vi "getVariableStatus.vi"(0 "Controller in":refnum<class "_Controller.lvclass">, 2 "var_number":u16, 5 "error in (no error)":errorcluster) -> (14 "Controller out":refnum<class "_Controller.lvclass">, 16 "var_value":string, 19 "error out":errorcluster)   [LabVIEW 2020, in "classes.lvlib" / "_Controller.lvclass"]
doc: "Retrieves the Variable Value (output) at the given Variable Number (input)\n\nProduced By:\n\n<B>Kod Integrations, LLC</B>\n4835 Marianne Drive\nMount Airy, MD 21771\nhttp://www.kodintegrations.com\nemail: info@kodintegrations.com\nphone: (240) 687-1288"
uses:
  _Controller.lvclass
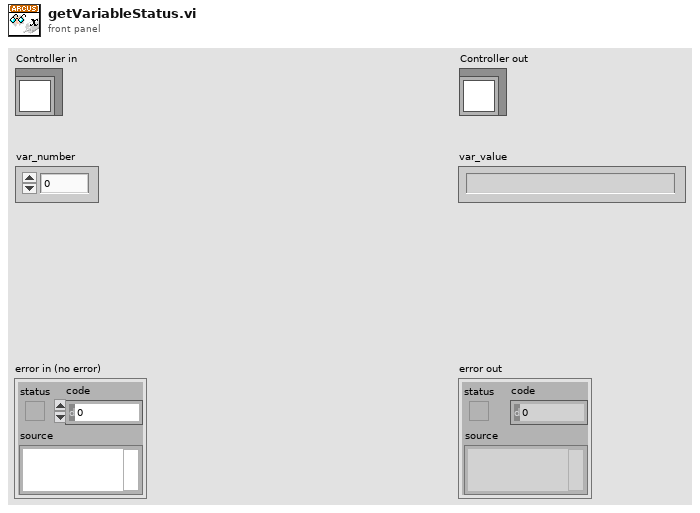
[diagram p1: front panel]
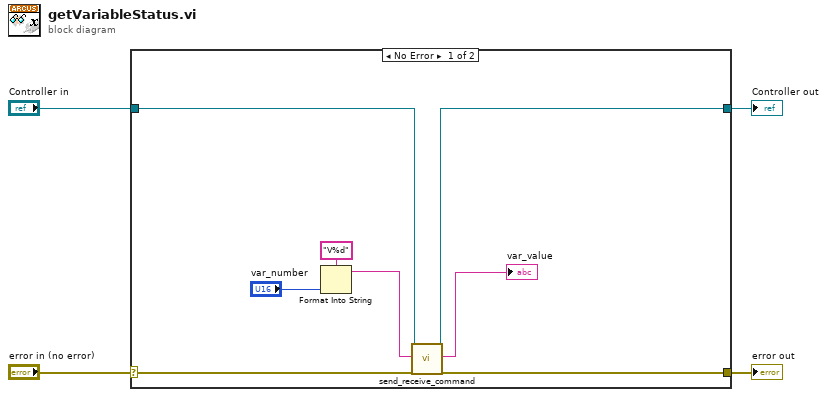
[diagram p0: block diagram]
diagram:
  n1 = case shown="No Error" "error in (no error)" {
    selector: "error in (no error)" -> [w12 w14]
    tunnel: [w11 w14] -> w3
    tunnel: [w9 w13] -> w1
    tunnel: "Controller in" -> [w10 w13]
    frame No Error {
      n2 = Format Into String(format string="V%d", "var_number") -> (resulting string=w6:string)  [unwired: 2 in, 1 out]
      n3 = call "send_receive_command.vi"("reference (in)"=w10, "ASCII Command (in)"=w6, "error in (no error)"=w12) -> ("reference (out)"=w9:refnum<class "_Controller.lvclass">, "response (out)"=→"var_value":string, "error out"=w11:errorcluster)  [unwired: 12 in, 2 out]
    }
    frame Error {
    }
  }
  "error out" <- w3
  "Controller out" <- w1
